vi "Theta 4.vi"(7 "XYZ_6012":dbl[](array[numeric])=[0.0, 0.0, 0.0], 11 "6R Type 2 Serial Arm Class in":refnum<class "NI_Robotics_6R Type 2 Serial Arm Class.lvclass">) -> (1 "Valid":bool, 2 "theta_4 array":dbl[](array[numeric]), 3 "6R Type 2 Serial Arm Class out":refnum<class "NI_Robotics_6R Type 2 Serial Arm Class.lvclass">)   [LabVIEW 2017, in "NI_Robotics_6R Type 2 Serial Arm Class.lvclass"]
uses:
  <vilib>/robotics/Kinematics/Analytical/6R/Type 2/NI_Robotics_6R Type 2 Serial Arm Class.lvclass
  c:/Program Files (x86)/National Instruments/LabVIEW 2017/vi.lib/robotics/Kinematics/Analytical/Generic/NI_Robotics_Analytical Serial Arm Class.lvclass
  <vilib>/robotics/Kinematics/Link/NI_Robotics_Link.lvclass/NI_Robotics_Link.ctl
  <vilib>/robotics/Kinematics/Link/Get Kinematic Parameters.vi
  <vilib>/robotics/Kinematics/Analytical/Generic/NI_Robotics_Analytical Serial Arm Class.lvclass
  c:/Program Files (x86)/National Instruments/LabVIEW 2017/vi.lib/robotics/Kinematics/Robot/NI_Robotics_Serial Robot Arm.lvclass
  <vilib>/robotics/Kinematics/Analytical/Generic/Accessors/Read alpha_n0.vi
  <vilib>/robotics/Kinematics/Robot/Get Links.vi
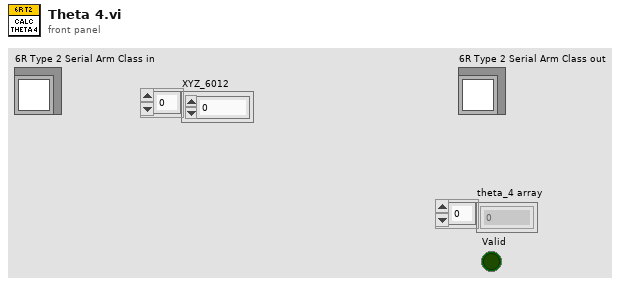
[diagram p1: front panel]
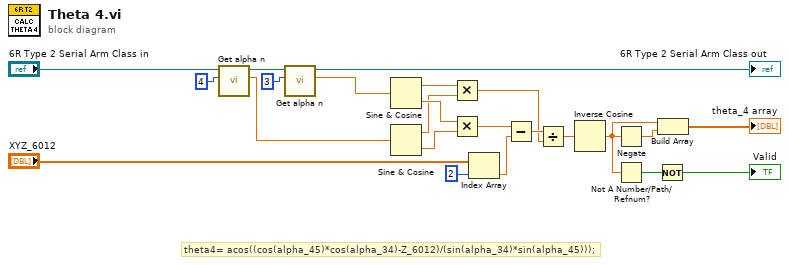
[diagram p0: block diagram]
diagram:
  # "theta4= acos((cos(alpha_45)*cos(alpha_34)-Z_6012)/(sin(alpha_34)*sin(alpha_45)));"
  n1 = call <vilib>:"Get alpha n.vi"("n"=4, "Analytical Serial Arm Class in"="6R Type 2 Serial Arm Class in") -> ("alpha n"=w19:dbl, "Analytical Serial Arm Class out"=w22:refnum<class "NI_Robotics_6R Type 2 Serial Arm Class.lvclass">)  [unwired: 8 in]
  n2 = call <vilib>:"Get alpha n.vi"("n"=3, "Analytical Serial Arm Class in"=w22) -> ("alpha n"=w18:dbl, "Analytical Serial Arm Class out"=→"6R Type 2 Serial Arm Class out":refnum<class "NI_Robotics_6R Type 2 Serial Arm Class.lvclass">)  [unwired: 8 in]
  n3 = Sine & Cosine(0:w18) -> (1:w10:dbl, 2:w15:dbl)
  n4 = Sine & Cosine(0:w19) -> (1:w11:dbl, 2:w14:dbl)
  n5 = Multiply(x=w10, y=w11) -> (x*y=w8:dbl)
  n6 = Multiply(x=w15, y=w14) -> (x*y=w12:dbl)
  n7 = Index Array(array="XYZ_6012", index=2) -> (element=w13:dbl)
  n8 = Subtract(x=w12, y=w13) -> (x-y=w9:dbl)
  n9 = Divide(x=w9, y=w8) -> (x/y=w5:dbl)
  n10 = Inverse Cosine(1:w5) -> (0:w2:dbl)
  n11 = Negate(x=w2) -> (-x=w6:dbl)
  n12 = Not A Number/Path/Refnum?(number/path/refnum=w2) -> (NaN/Path/Refnum?=w3:bool)
  n13 = Not(x=w3) -> (.not. x?=→"Valid":bool)
  n14 = Build Array(w2, w6) -> (→"theta_4 array":dbl[])
